vi "DIO64 OpenResource.vi"(0 "board in":u16 format="%.0x", 1 "resourceName":string, 5 "base IO":u16=384 format="%.0x", 11 "error in (no error)":errorcluster) -> (4 "board out":u16 format="%.0x", 15 "error out":errorcluster)   [LabVIEW 2012]
doc: "DIO64 Open initializes the selected DIO-64 board.\n\nCopyright (c) 2002 Viewpoint Systems Inc. All Rights Reserved"
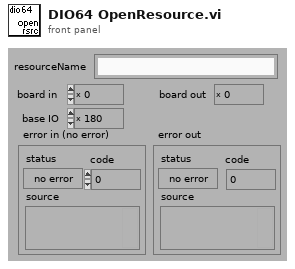
[diagram p1: front panel]
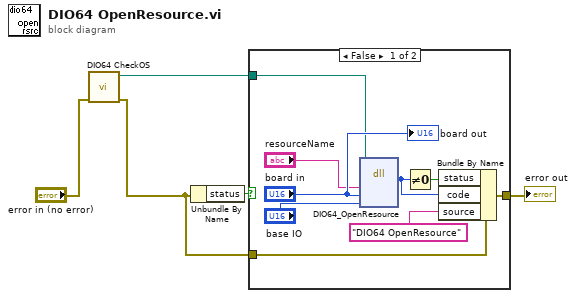
[diagram p0: block diagram]
diagram:
  n1 = call "DIO64 CheckOS.vi"("error in"="error in (no error)") -> ("error out"=w2:errorcluster, "path in"=w1:path)  [unwired: 9 in]
  n2 = Unbundle By Name(w2) -> ("status"=w5:bool)
  n3 = case shown="False" w5 {
    tunnel: w2 -> [w12 w15]
    tunnel: [w11 w15] -> w4
    tunnel: w1 -> [w6 _]
    frame False {
      n4 = dll-call lib="C:/Users/EDM/Desktop/experiment control/subvis/DIO64/DIO64_Visa32.dll" fn="DIO64_OpenResource"(path in=w6, "resourceName"="resourceName", "board"="board in", "baseio"="base IO") -> ("return type"=w14:i32)  [unwired: 5 in, 2 out]
      n5 = Not Equal To 0?(x=w14) -> (x != 0?=w13:bool)
      n6 = Bundle By Name(cluster=w12, "status"=w13, "code"=w14, "source"="DIO64 OpenResource") -> (w11:errorcluster)
      "board out" <- "board in"
    }
    frame True {
    }
  }
  "error out" <- w4
